vi "ReportError.vi"(8 "error in (no error)":errorcluster, 9 "Additional Info":string, 10 "ErrorReported":errorcluster, 11 "ModuleID":i32) -> (0 "error out":errorcluster)   [LabVIEW 2014, in "ScopeModule.lvlib"]
uses:
  ScopeModule.lvlib
  PublicAPI/Arguments/Broadcasts/clErrorRpt.ctl
  clEventType.ctl
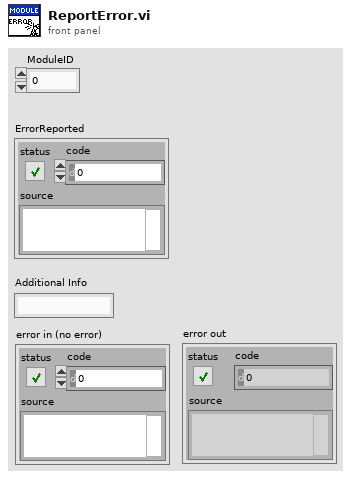
[diagram p1: front panel]
types:
  T1 = typedef "ScopeModule.lvlib/clEventType.ctl" = cluster{"ModuleID":i32, "Data":variant}
  T2 = typedef "ScopeModule.lvlib/clErrorRpt.ctl" = cluster{"error":errorcluster, "AdditionalInfo":string}
  T3 = typedef "ScopeModule.lvlib/clBroadcastEvents.ctl" = cluster{"DidInit":refnum<user-event>, "StatusUpdate":refnum<user-event>, "ErrorReport":refnum<user-event>, "DidStop":refnum<user-event>, "PathToINI":refnum<user-event>}
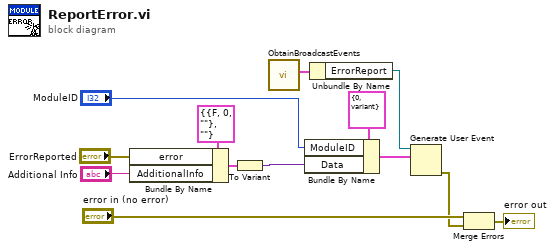
[diagram p0: block diagram]
diagram:
  n1 = Bundle By Name(cluster=T2 {"error"={"status"=FALSE, "code"=0, "source"=""}, "AdditionalInfo"=""} ("Cluster"), "error"="ErrorReported", "AdditionalInfo"="Additional Info") -> (w10:T2)
  n2 = To Variant(anything=w10) -> (Variant=w8:variant)
  n3 = call "ObtainBroadcastEvents.vi"() -> ("clBroadcastEvents"=w6:T3)  [unwired: 10 in, 1 out]
  n4 = Bundle By Name(cluster=T1 {"ModuleID"=0, "Data"=variant} ("clEventType"), "ModuleID"="ModuleID", "Data"=w8) -> (w5:T1)
  n5 = Unbundle By Name(w6) -> ("ErrorReport"=w4:refnum<user-event>)
  n6 = Generate User Event(user event=w4, event data cluster=w5) -> (error out=w1:errorcluster)  [unwired: 2 in, 1 out]
  n7 = Merge Errors("error in (no error)", w1) -> (→"error out":errorcluster)
